vi "RichToFlatnixnet_grpc_StartRequest.vi"(5 "OutputClusterType":T1, 11 "InputCluster":T4) -> (3 "OutputCluster":T1)   [LabVIEW 2025, in "xnet-grpc_client.lvlib"]
uses:
  xnet-grpc_client.lvlib
  nixnet_grpc_StartRequest.ctl
  nixnet_grpc_StartRequest_scope_enum/nixnet_grpc_StartRequest_scope_enum.lvclass
  nidevice_grpc_Session.ctl
  nixnet_grpc_StartRequest_Flat.ctl
  nidevice_grpc_Session_Flat.ctl
  nixnet_grpc_StartStopScope.ctl
  nixnet_grpc_StartRequest_scope_enum/nixnet_grpc_StartRequest_scope_enum.lvclass/nixnet_grpc_StartRequest_scope_enum.ctl
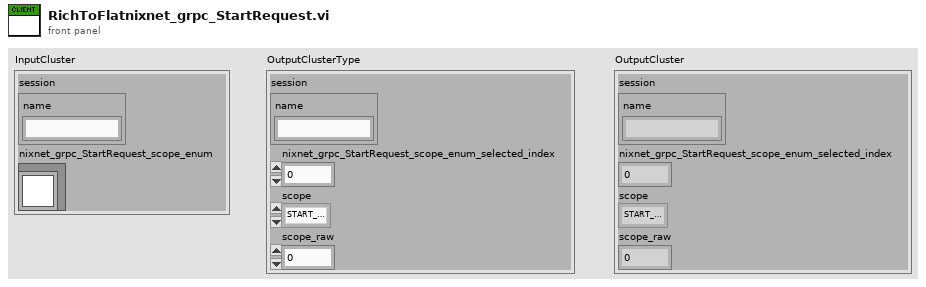
[diagram p1: front panel]
types:
  T1 = typedef "xnet-grpc_client.lvlib/nixnet_grpc_StartRequest_Flat.ctl" = cluster{"session":T2, "nixnet_grpc_StartRequest_scope_enum_selected_index":i32, "scope":T3, "scope_raw":u32}
  T2 = typedef "xnet-grpc_client.lvlib/nidevice_grpc_Session_Flat.ctl" = cluster{"name":string}
  T3 = typedef "xnet-grpc_client.lvlib/nixnet_grpc_StartStopScope.ctl" = enum32{"START_STOP_SCOPE_NORMAL", "START_STOP_SCOPE_SESSION_ONLY", "START_STOP_SCOPE_INTERFACE_ONLY", "START_STOP_SCOPE_SESSION_ONLY_BLOCKING"}
  T4 = typedef "xnet-grpc_client.lvlib/nixnet_grpc_StartRequest.ctl" = cluster{"session":T5, "nixnet_grpc_StartRequest_scope_enum":refnum<class "nixnet_grpc_StartRequest_scope_enum.lvclass">}
  T5 = typedef "xnet-grpc_client.lvlib/nidevice_grpc_Session.ctl" = cluster{"name":string}
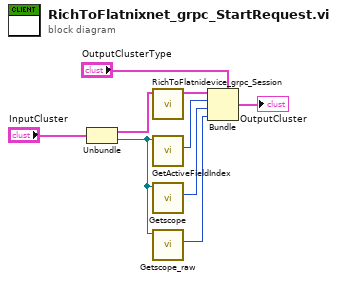
[diagram p0: block diagram]
diagram:
  n1 = Unbundle "Unbundle"("InputCluster") -> ("session"=w6:T5, "nixnet_grpc_StartRequest_scope_enum"=w4:refnum<class "nixnet_grpc_StartRequest_scope_enum.lvclass">)
  n2 = call "RichToFlatnidevice_grpc_Session.vi"("InputCluster"=w6) -> ("OutputCluster"=w5:T2)  [unwired: 10 in]
  n3 = call "GetActiveFieldIndex.vi"("OneOfTemplate in"=w4) -> ("Active Field Index"=w3:i32)  [unwired: 8 in, 2 out]
  n4 = call "Getscope.vi"("OneOfTemplate in"=w4) -> ("Get_Val"=w2:T3)  [unwired: 8 in, 2 out]
  n5 = call "Getscope_raw.vi"("OneOfTemplate in"=w4) -> ("Get_Val"=w1:u32)  [unwired: 8 in, 2 out]
  n6 = Bundle "Bundle"(cluster="OutputClusterType", "session"=w5, "nixnet_grpc_StartRequest_scope_enum_selected_index"=w3, "scope"=w2, "scope_raw"=w1) -> (→"OutputCluster":T1)
